vi "W9EO82,FBO8PP_2 .vi"() -> ()   [LabVIEW 2021]
panel:
  out "String":string
  in  "Slide":i32(slide) scale=0.0..2.0
  out "Eredmény":dbl
  in  "Numeric":dbl
  out "gomb":bool
  in  "kapcsoló":bool
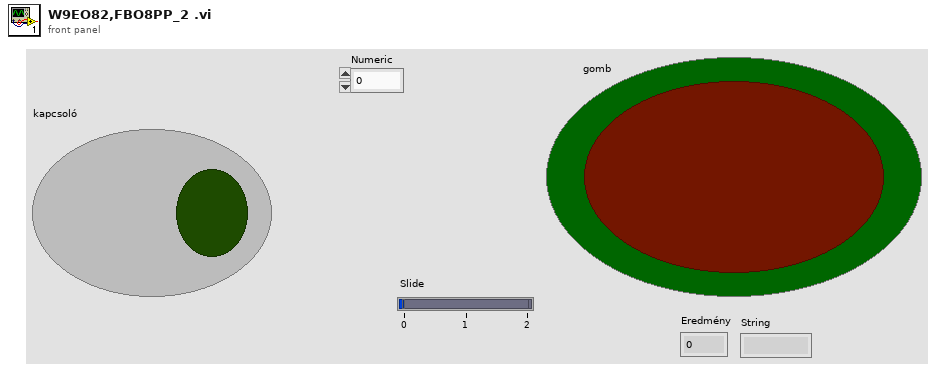
[diagram p1: front panel]
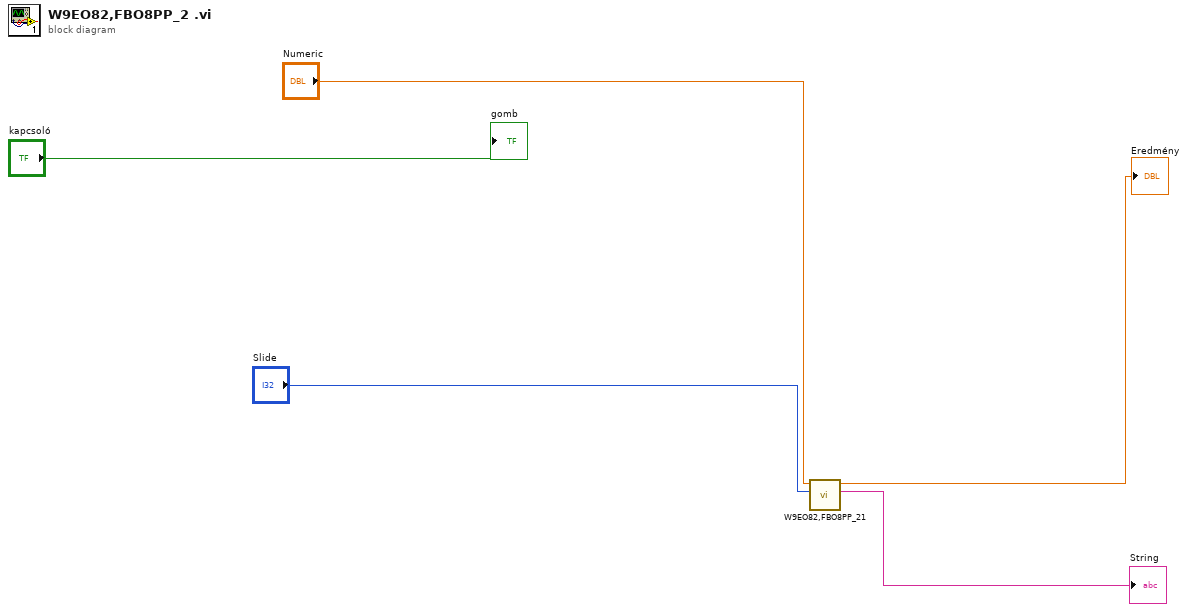
[diagram p0: block diagram]
diagram:
  n1 = call "W9EO82,FBO8PP_21.vi"("Slide"="Slide", "Numeric in"="Numeric") -> ("String"=→"String":string, "Numeric out"=→"Eredmény":dbl)  [unwired: 8 in]
  "gomb" <- "kapcsoló"
